vi "Lim_FileClose.vi"(8 "error in (no error)":errorcluster, 11 "hFile in":T1) -> (0 "error out":errorcluster, 2 "LIMRESULT":i16)   [LabVIEW 2014, in "ND2_Reader_32.lvlib"]
uses:
  ND2_Reader_32.lvlib
  controls/numeric_LIMFILEHANDLE.ctl
  nd2 reader/SDK/bin/x86/v6_w32_nd2ReadSDK.dll
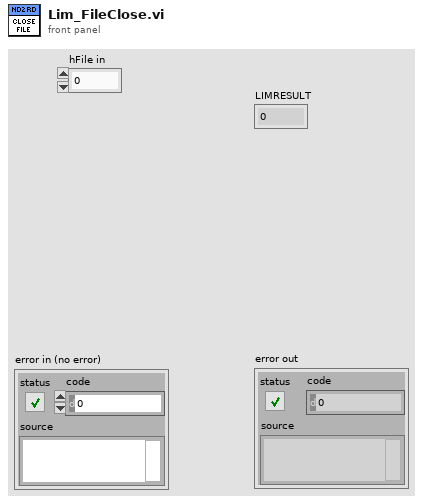
[diagram p1: front panel]
types:
  T1 = typedef "numeric_LIMFILEHANDLE.ctl" = i32
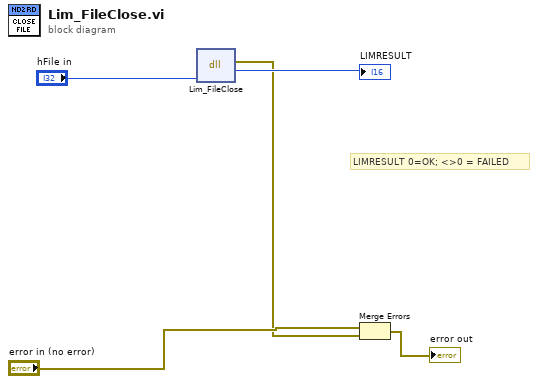
[diagram p0: block diagram]
diagram:
  # "LIMRESULT 0=OK; <>0 = FAILED"
  n1 = dll-call lib="C:/Users/VirtualUser/Desktop/EPA-Vision/EPA Image Source LV2014 2.0.0 2016-02-23/ND2_Reader_32bit/nd2 reader/SDK/bin/x86/v6_w32_nd2ReadSDK.dll" fn="Lim_FileClose"("hFile"="hFile in") -> (error out=w2:errorcluster, "LIMRESULT"=→"LIMRESULT":i16)  [unwired: 3 in, 2 out]
  n2 = Merge Errors("error in (no error)", w2) -> (→"error out":errorcluster)
